vi "getREF.vi"(8 "error in (no error)":errorcluster, 11 "Instrument.LockinAPI in":refnum<class "Instrument.LockinAPI.lvclass">) -> (0 "error out":errorcluster, 2 "REFconfig":T1[](array[typedef]), 3 "Instrument.LockinAPI out":refnum<class "Instrument.LockinAPI.lvclass">)   [LabVIEW 2019, in "Instrument.LockinAPI.lvclass"]
doc: "API to get the results of lockin calculation.\n\nIf address=\"\", this API reads from localhost\nIf address is remote lockin, you need to add this computer to allowed whitelist on the lockin computer you are trying to access."
uses:
  Instrument.LockinAPI.lvclass
  C:/Users/patrick/Documents/GitHub/Instrument-Framework/lvsrc/Instrument/Instrument.lvclass
  Typedefs/LockinAPI.REFconfig--Cluster.ctl
  Typedefs/LockinAPI.Commands--Enum.ctl
  b5ba668f-388a-4953-9e5e-5fc2c5d58124.vi
  b5ba668f-388a-4953-9e5e-5fc2c5d58124.vi/15e01d63-4acf-49b6-9d01-c6bc6fca5d96.vi
  b5ba668f-388a-4953-9e5e-5fc2c5d58124.vi/15e01d63-4acf-49b6-9d01-c6bc6fca5d96.vi/9bf26c14-7a1e-44c4-b716-0bb6d7dcfc7d.vi
  b5ba668f-388a-4953-9e5e-5fc2c5d58124.vi/15e01d63-4acf-49b6-9d01-c6bc6fca5d96.vi/e5ed59a6-19ee-421d-a916-1f75e2973094.vi
  Instrument/Protected/Validate API method.vi
  Instrument/Private/Get RC Connection Status.vi
  Instrument/API/Send and Receive.vi
  <vilib>/Utility/Data Type/Get Type Information.vi
  <vilib>/JDP Science/JSONtext/JSON text to Variant.vi
  <vilib>/JDP Science/JSONtext/LVClass Serializer/JSONtext LVClass Serializer.lvclass
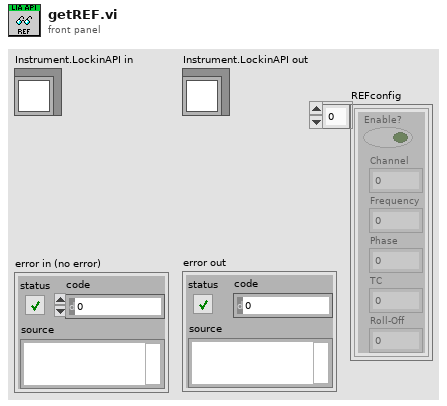
[diagram p1: front panel]
types:
  T1 = typedef "Instrument.LockinAPI.lvclass/LockinAPI.REFconfig--Cluster.ctl" = cluster{"Enable?":bool, "Channel":i32, "Frequency":dbl, "Phase":dbl, "TC":dbl, "Roll-Off":i32}
  T2 = typedef "Instrument.LockinAPI.lvclass/LockinAPI.Commands--Enum.ctl" = enum16{"setAI", "setAO", "setAO_Amplitude", "setAO_DC", "setAO_Frequency", "setAO_Phase", "setAO_Function", "setAO_I+", "setREF", "setREF_Frequency", "setREF_Phase", "setREF_TC", "setREF_Roll-Off", "setDAQ", "setSampling", "setOffset", "setState", "getState", "getAO", "getAI", "getResults", "getSampling", "getAOconfig", "getREFconfig", "setInputGain", "setOutputGain", "getInputGain", "getOutputGain", "setSamplingMode", "getSamplingMode", "setSweep", "setSweepTime", "setSweepTable", "getStatus", "getSweepResults", "getSweepWaveforms", "startSweep", "stopSweep", "setAUX", "getAUX"}
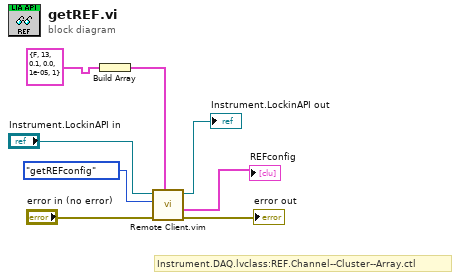
[diagram p0: block diagram]
diagram:
  # "Instrument.DAQ.lvclass:REF.Channel--Cluster--Array.ctl"
  n1 = Build Array(T1 {"Enable?"=FALSE, "Channel"=13, "Frequency"=0.1, "Phase"=0.0, "TC"=1e-05, "Roll-Off"=1} ("REFconfig")) -> (w1:T1[])
  n2 = call "Remote Client.vim"("Data Out type"=w1, "error in (no error)"="error in (no error)", "Command in"=LockinAPI.Commands--Enum."getREFconfig" ("Command"), "Instrument in"="Instrument.LockinAPI in") -> ("error out"=→"error out":errorcluster, "Data out"=→"REFconfig":T1[], "Instrument out"=→"Instrument.LockinAPI out":refnum<class "Instrument.LockinAPI.lvclass">)  [unwired: 4 in, 1 out]
